vi "createExperimentFolder.vi"(11 "Experiment Name":string) -> (3 "created path":path)   [LabVIEW 2013]
panel:
  out "error out":errorcluster
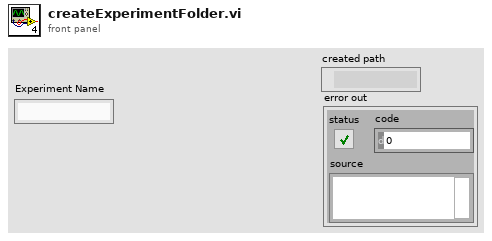
[diagram p1: front panel]
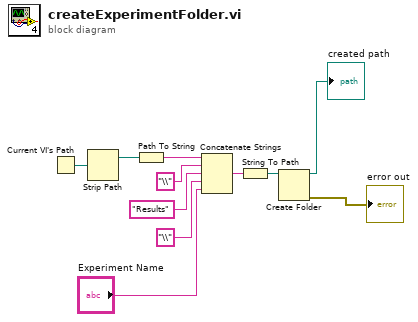
[diagram p0: block diagram]
diagram:
  n1 = Current VI's Path() -> (path=w8:path)
  n2 = Strip Path(path=w8) -> (stripped path=w9:path)  [unwired: 1 out]
  n3 = Path To String(path=w9) -> (string=w10:string)
  n4 = Concatenate Strings(w10, "\\" ("string"), "Results" ("string"), "\\" ("string"), "Experiment Name") -> (w7:string)
  n5 = String To Path(string=w7) -> (path=w6:path)
  n6 = Create Folder(path (use dialog)=w6) -> (created path=→"created path":path, error out=→"error out":errorcluster)  [unwired: 2 in, 1 out]
